vi "WZ5005E-Set Addr.vi"(8 "error in":errorcluster caption="错误输入（无错误）", 9 "修改地址":string="02", 10 "当前地址":string="01", 11 "MyIndex":u8) -> (0 "error out":errorcluster, 3 "Result":bool)   [LabVIEW 2015, in "WZ5005E.lvlib"]
uses:
  WZ5005E.lvlib
  <vilib>/Instr/_visa.llb/VISA Configure Serial Port (Instr).vi
panel:
  out "VISA":refnum<visa-resource-name>
  out "Send":string
  # "修改成功会把当前地址改为修改后的地址"
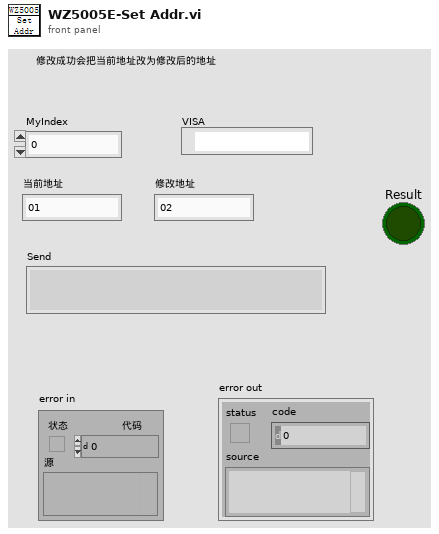
[diagram p1: front panel]
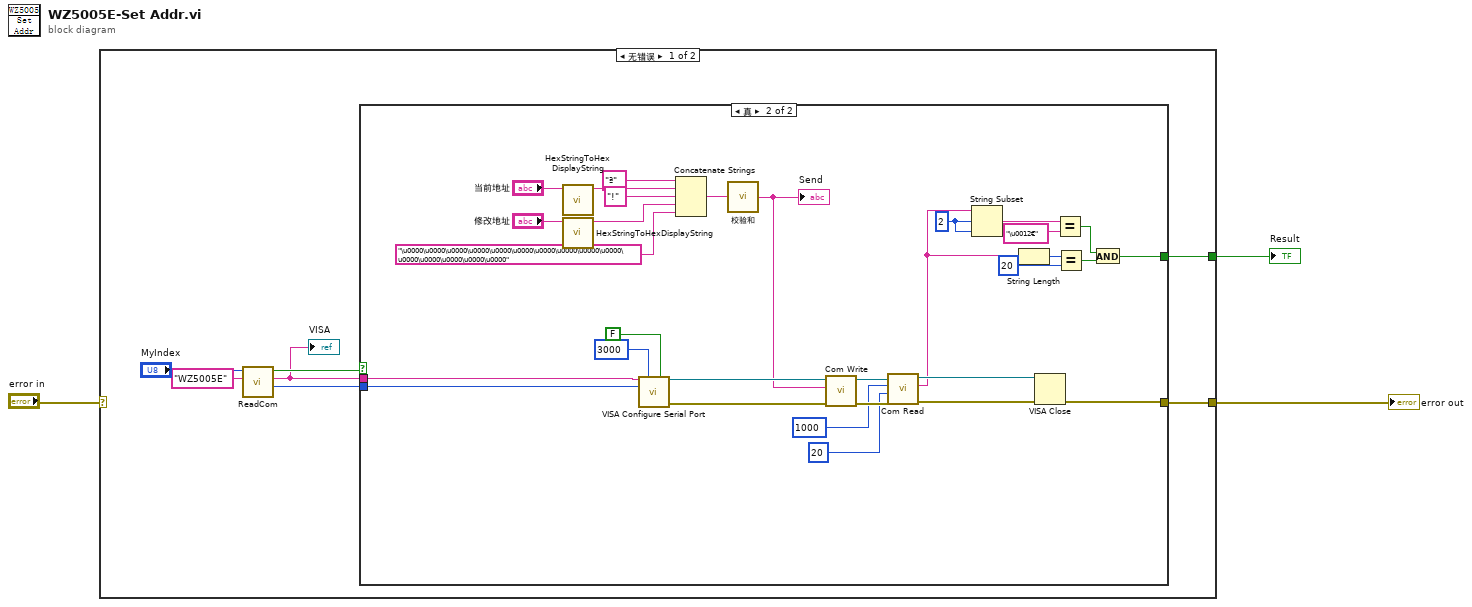
[diagram p0: block diagram]
diagram:
  n1 = case shown="无错误" "error in" {
    selector: "error in" -> [_ w42]
    tunnel: [w10 w42] -> w3
    tunnel: [w4 _] -> w1
    frame No Error {
      n2 = call "ReadCom.vi"("仪器名称"="WZ5005E", "MyIndex"="MyIndex") -> ("Baudrate"=w5:i32, "COM"=w6:string, "OK?"=w7:bool)  [unwired: 7 in]
      "VISA" <- w6
      n3 = case shown="真" w7 {
        tunnel: [_ w41] -> w10
        tunnel: w6 -> [_ w40]
        tunnel: w5 -> [_ w39]
        tunnel: [_ w21] -> w4
        frame False {
        }
        frame True {
          w28 = 2 ("偏移量(0)")
          n4 = call "HexStringToHexDisplayString.vi"("正常显示HEX字符串"="当前地址") -> ("HEX显示字符串"=w14:string)  [unwired: 10 in]
          n5 = call "HexStringToHexDisplayString.vi"("正常显示HEX字符串"="修改地址") -> ("HEX显示字符串"=w19:string)  [unwired: 10 in]
          n6 = call-poly "VISA Configure Serial Port"("VISA resource name"=w40, "timeout (10sec)"=u32 3000, "Enable Termination\nChar (T)"=FALSE ("Enable Termination\nChar (T)"), "baud rate (9600)"=w39) -> ("VISA resource name out"=w37:refnum<visa-resource-name>, "error out"=w36:errorcluster)  [unwired: 10 in]
          n7 = Concatenate Strings("ª", w14, "!", w19, "\u0000\u0000\u0000\u0000\u0000\u0000\u0000\u0000\u0000\u0000\u0000\u0000\u0000\u0000\u0000") -> (w17:string)
          n8 = call "校验和.vi"("输入（Hex）"=w17) -> ("输出"=w11:string)
          "Send" <- w11
          n9 = call "Com Write.vi"("错误输入（无错误）"=w36, "Wbuff"=w11, "VISA In"=w37) -> ("错误输出"=w34:errorcluster, "VISA Out"=w35:refnum<visa-resource-name>)  [unwired: 6 in, 1 out]
          n10 = call "Com Read.vi"("错误输入（无错误）"=w34, "num"=u32 20, "超时"=u32 1000, "VISA In"=w35) -> ("错误输出"=w33:errorcluster, "buff"=w22:string, "VISA Out"=w32:refnum<visa-resource-name>)  [unwired: 4 in, 1 out]
          n11 = String Subset(string=w22, offset (0)=w28, length (rest)=w28) -> (substring=w27:string)
          n12 = String Length(string=w22) -> (length=w23:i32)
          n13 = VISA Close(VISA resource name=w32, error in (no error)=w33) -> (error out=w41:errorcluster)
          n14 = Equal?(x=w27, y="\u0012€" ("正则表达式")) -> (x = y?=w29:bool)
          n15 = Equal?(x=w23, y=20) -> (x = y?=w25:bool)
          n16 = And(x=w29, y=w25) -> (x .and. y?=w21:bool)
        }
      }
    }
    frame Error {
    }
  }
  "error out" <- w3
  "Result" <- w1
